vi "Drive Straight Pigeon.vi"(4 "D Gain":dbl=5e-05 format="%#_13g", 6 "P Gain":dbl=0.0725 format="%#_13g", 9 "Buttons":bool[](array[boolean]), 10 "Axes":dbl[](array[numeric]), 11 "Get All":T2 {"Calibration"."CurrentMode" items=["BootTareGryoAccel"=0, "Temperature"=1, "Magnetometer12Pt"=2, "Magnetometer360"=3, "Accelerometer"=5]}) -> (2 "Left Motor Value":dbl, 3 "Right Motor Value":dbl, 5 "Control Mode":T1)   [LabVIEW 2016]
uses:
  <vilib>/Rock Robotics/WPI/ThirdParty/Sensors/Pigeon IMU/CTRE_PigeonIMU_GlobalStatus.ctl
  <vilib>/Rock Robotics/WPI/ThirdParty/Sensors/Pigeon IMU/CTRE_PigeonIMU_PigeonState.ctl
  <vilib>/Rock Robotics/WPI/ThirdParty/Sensors/Pigeon IMU/CTRE_PigeonIMU_CalibrationMode.ctl
  <vilib>/Rock Robotics/WPI/ThirdParty/CanMotor/TalonSRX/WPI_CANTalonSRX_APIControlMode.ctl
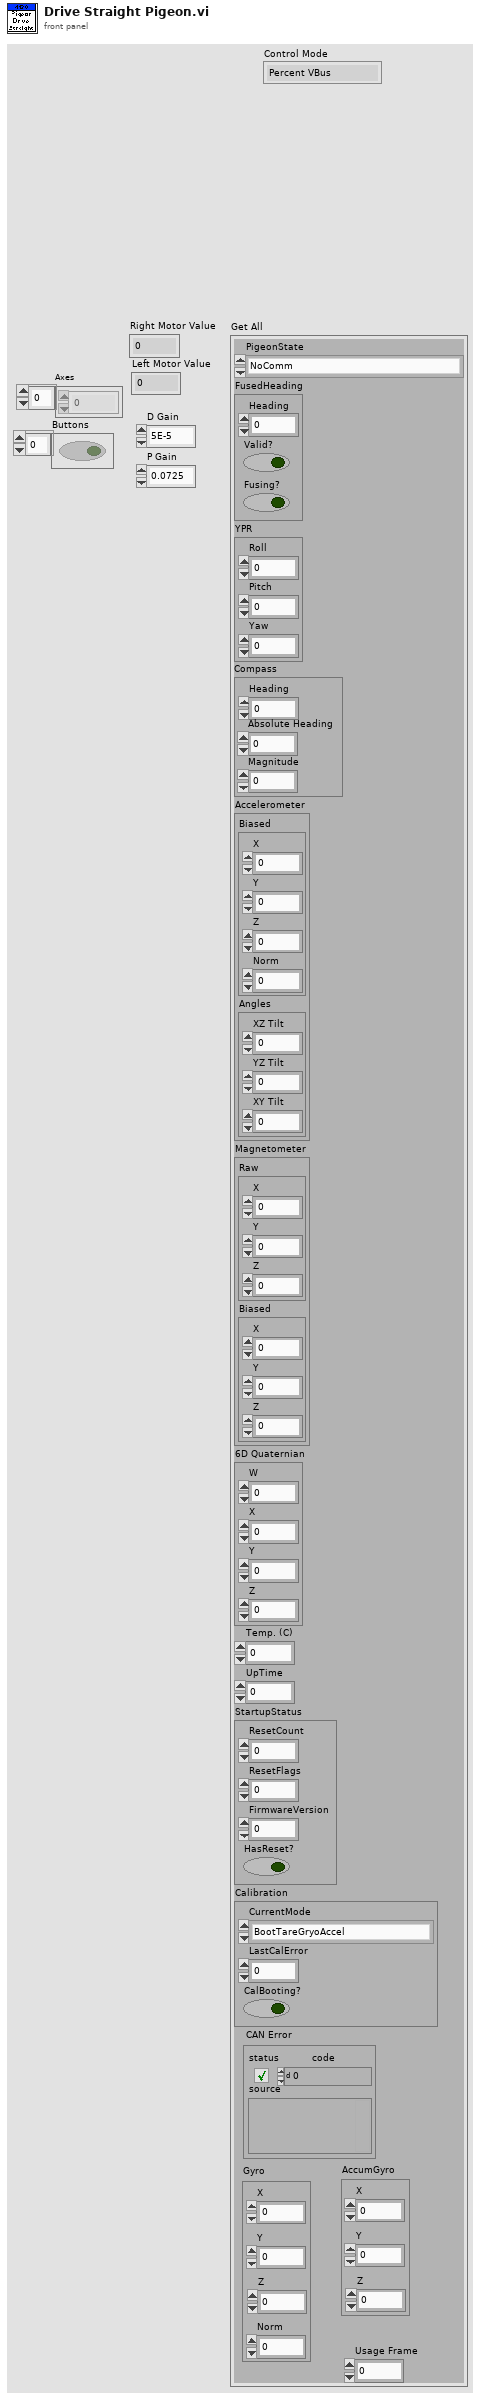
[diagram p1: front panel]
types:
  T1 = typedef "WPI_CANTalonSRX_APIControlMode.ctl" = enum8{"Percent VBus", "Speed", "Position", "Slave", "Unchanged / Invalid", "Voltage Compensation", "Current", "Motion Profile", "Motion Magic"}
  T2 = typedef "CTRE_PigeonIMU_GlobalStatus.ctl" = cluster{"PigeonState":T3, "FusedHeading":cluster{"Heading":dbl, "Valid?":bool, "Fusing?":bool}, "YPR":cluster{"Yaw":dbl, "Pitch":dbl, "Roll":dbl}, "Compass":cluster{"Heading":dbl, "Magnitude":dbl, "Absolute Heading":dbl}, "Accelerometer":cluster{"Biased":cluster{"X":i16, "Y":i16, "Z":i16, "Norm":i16}, "Angles":cluster{"XZ Tilt":dbl, "YZ Tilt":dbl, "XY Tilt":dbl}}, "Magnetometer":cluster{"Raw":cluster{"X":i16, "Y":i16, "Z":i16}, "Biased":cluster{"X":i16, "Y":i16, "Z":i16}}, "Gyro":cluster{"X":dbl, "Y":dbl, "Z":dbl, "Norm":dbl}, "6D Quaternian":cluster{"W":dbl, "X":dbl, "Y":dbl, "Z":dbl}, "Temp. (C)":dbl, "UpTime":u32, "StartupStatus":cluster{"ResetCount":i32, "ResetFlags":i32, "FirmwareVersion":i32, "HasReset?":bool}, "Calibration":cluster{"CurrentMode":T4, "LastCalError":i32, "CalBooting?":bool}, "CAN Error":errorcluster, "AccumGyro":cluster{"X":dbl, "Y":dbl, "Z":dbl}, "Usage Frame":u32}
  T3 = typedef "CTRE_PigeonIMU_PigeonState.ctl" = enum16{"NoComm", "Initializing", "Ready", "UserCalibration"}
  T4 = typedef "CTRE_PigeonIMU_CalibrationMode.ctl" = u16
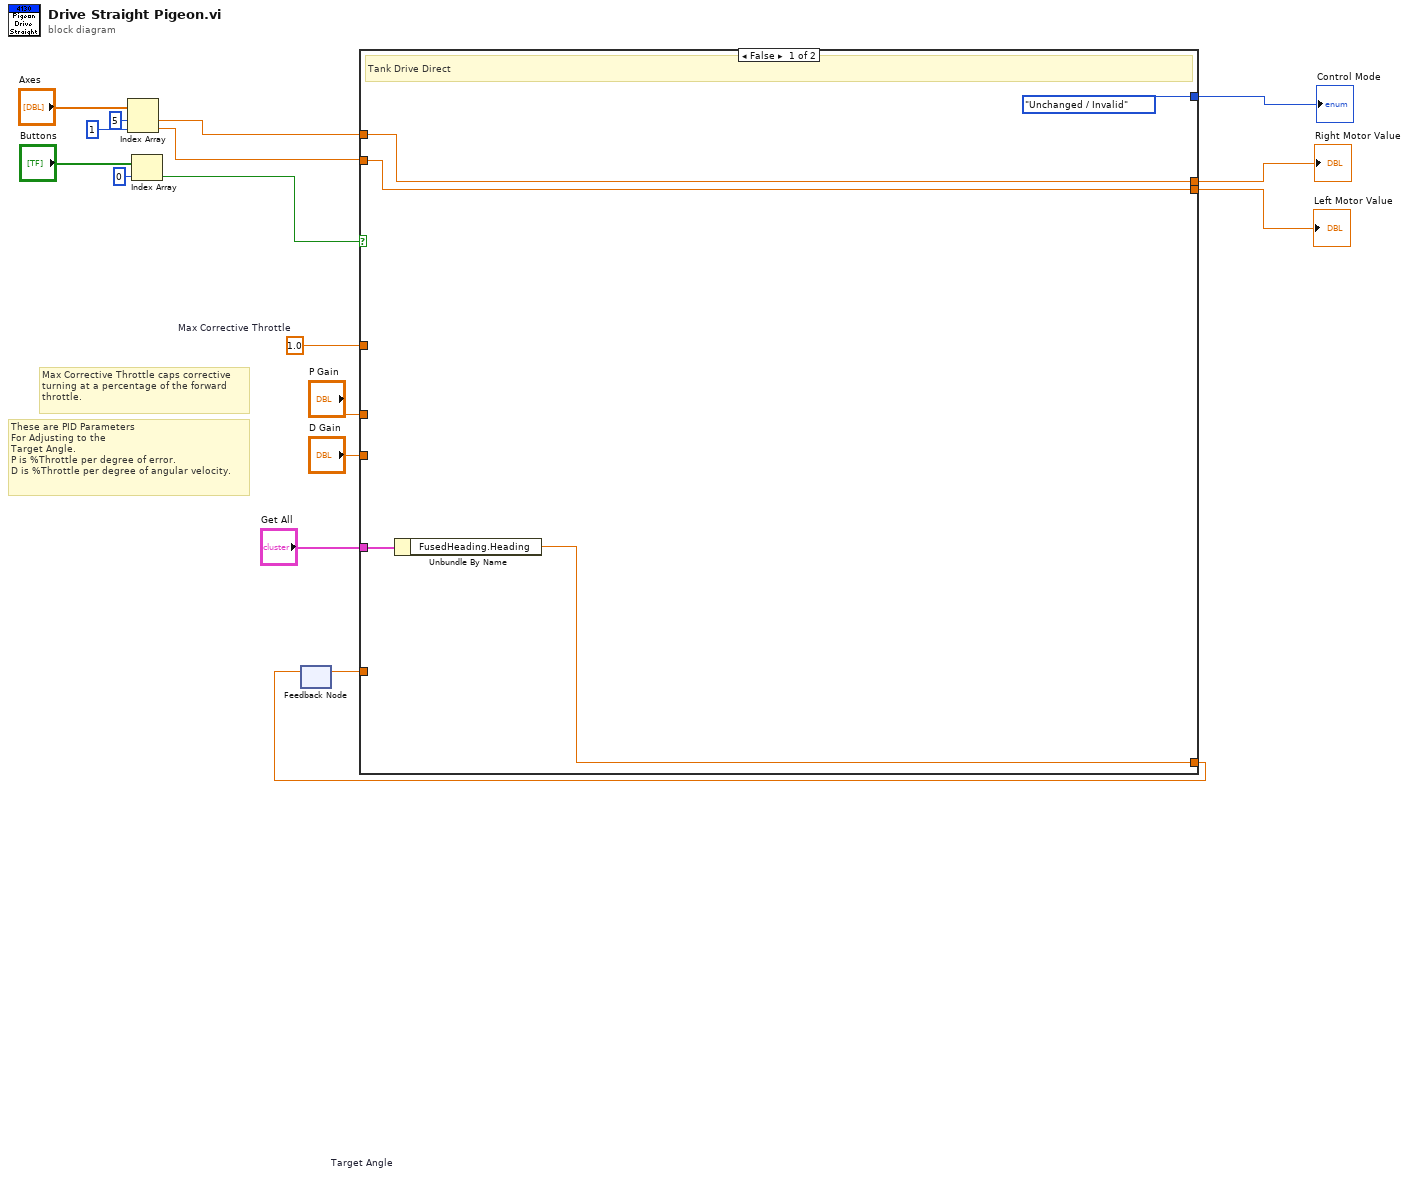
[diagram p0: block diagram]
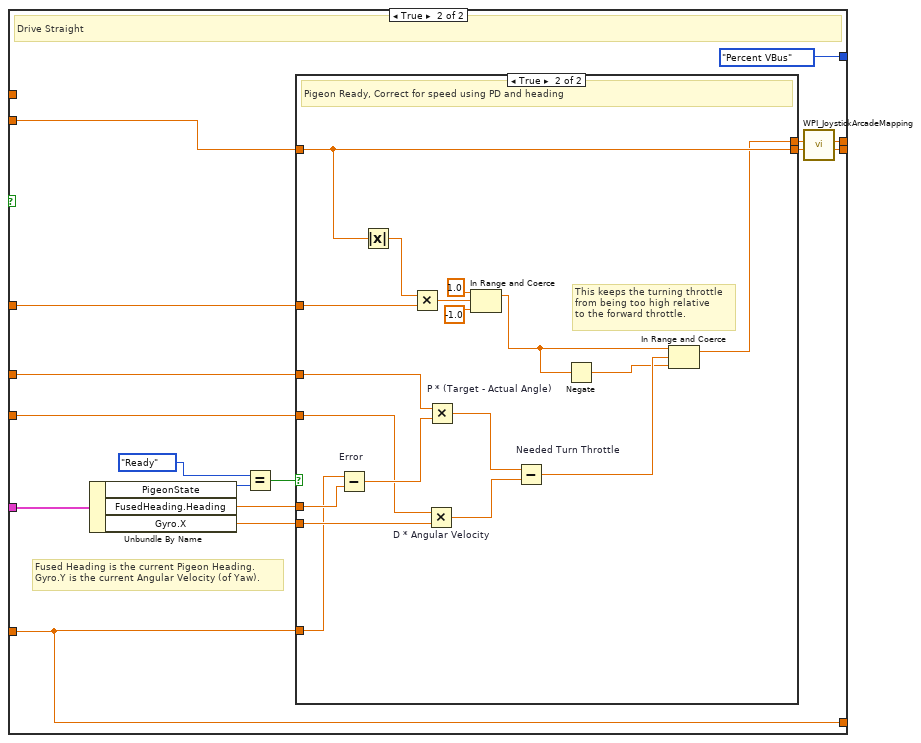
[diagram p2: hidden frame]
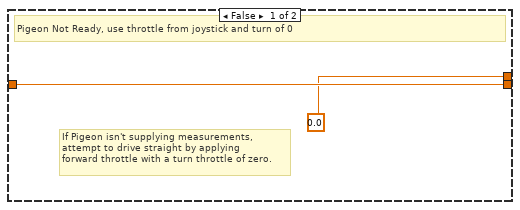
[diagram p3: hidden frame]
diagram:
  w14 = 1.0  # Max Corrective Throttle
  # "Max Corrective Throttle caps corrective\nturning at a percentage of the forward\nthrottle."
  # "These are PID Parameters\nFor Adjusting to the\nTarget Angle.\nP is %Throttle per degree of error.\nD is %Throttle per degree of angular velocity."
  n1 = Index Array(array="Axes", index #1=5 ("index"), index #2=1 ("index")) -> (element #1=w5:dbl, element #2=w4:dbl)
  n2 = Index Array(array="Buttons", index=0) -> (element=w3:bool)
  n3 = feedback #1 "Target Angle"() -> (w15:dbl)  [unwired: 1 in]
  n4 = case shown="False" w3 {
    tunnel: w5 -> [w19 _]
    tunnel: w4 -> [w18 w37]
    tunnel: "P Gain" -> [_ w32]
    tunnel: "D Gain" -> [_ w31]
    tunnel: [w22 w24] -> w13
    tunnel: w15 -> [_ w24]
    tunnel: w14 -> [_ w30]
    tunnel: [w19 w27] -> w12
    tunnel: [w18 w26] -> w11
    tunnel: "Get All" -> [w21 w25]
    tunnel: [WPI_CANTalonSRX_APIControlMode."Unchanged / Invalid" ("Control Mode") WPI_CANTalonSRX_APIControlMode."Percent VBus" ("Control Mode")] -> w1
    frame False {
      # "Tank Drive Direct"
      n5 = Unbundle By Name(w21) -> ("FusedHeading.Heading"=w22:dbl)
    }
    frame True {
      # "Fused Heading is the current Pigeon Heading.\nGyro.Y is the current Angular Velocity (of Yaw)."
      # "Drive Straight"
      n6 = Unbundle By Name(w25) -> ("PigeonState"=w35:T3, "FusedHeading.Heading"=w34:dbl, "Gyro.X"=w33:dbl)
      n7 = Equal?(x=CTRE_PigeonIMU_PigeonState."Ready" ("PigeonState"), y=w35) -> (x = y?=w38:bool)
      n8 = case shown="True" w38 {
        tunnel: w37 -> [w40 w49]
        tunnel: [w40 w49] -> w28
        tunnel: [0.0 ("upper limit") w42] -> w29
        tunnel: w34 -> [_ w58]
        tunnel: w24 -> [_ w41]
        tunnel: w33 -> [_ w55]
        tunnel: w32 -> [_ w56]
        tunnel: w31 -> [_ w54]
        tunnel: w30 -> [_ w51]
        frame False {
          # "If Pigeon isn't supplying measurements,\nattempt to drive straight by applying\nforward throttle with a turn throttle of zero."
          # "Pigeon Not Ready, use throttle from joystick and turn of 0"
        }
        frame True {
          # "This keeps the turning throttle\nfrom being too high relative\nto the forward throttle."
          # "Pigeon Ready, Correct for speed using PD and heading"
          n9 = Subtract "Error"(x=w41, y=w58) -> (x-y=w57:dbl)
          n10 = Absolute Value(x=w49) -> (abs(x)=w50:dbl)
          n11 = Multiply ("P * (Target - Actual Angle)")(x=w50, y=w51) -> (x*y=w46:dbl)
          n12 = Multiply "D * Angular Velocity"(x=w54, y=w55) -> (x*y=w52:dbl)
          n13 = Multiply "P * (Target - Actual Angle)"(x=w56, y=w57) -> (x*y=w53:dbl)
          n14 = In Range and Coerce(upper limit=1.0, x=w46, lower limit=-1.0) -> (coerced(x)=w44:dbl)  [unwired: 1 out]
          n15 = Subtract "Needed Turn Throttle"(x=w53, y=w52) -> (x-y=w45:dbl)
          n16 = Negate(x=w44) -> (-x=w43:dbl)
          n17 = In Range and Coerce(upper limit=w44, x=w45, lower limit=w43) -> (coerced(x)=w42:dbl)  [unwired: 1 out]
        }
      }
      n18 = call <vilib>:"WPI_JoystickArcadeMapping.vi"("Y axis value"=w28, "X axis value"=w29) -> ("Right Motor Value"=w26:dbl, "Left Motor Value"=w27:dbl)  [unwired: 8 in]
    }
  }
  "Right Motor Value" <- w12
  "Left Motor Value" <- w11
  "Control Mode" <- w1
  n19 = feedback-in #1(w13) -> ()
